vi "New 4ch.vi"(0 "VISA resource name out":refnum<visa-resource-name>, 9 "Number of channels":i32, 11 "error out":errorcluster) -> (3 "VISA resource name out 2":refnum<visa-resource-name>, 4 "element":dbl, 6 "element 2":dbl, 8 "element 3":dbl, 10 "element 4":dbl, 15 "error out 2":errorcluster)   [LabVIEW 2015]
uses:
  <instrlib>/Keithley 27XX/Public/Data/Read Multiple Direct.vi
  <instrlib>/Keithley 27XX/Keithley 27XX.lvlib
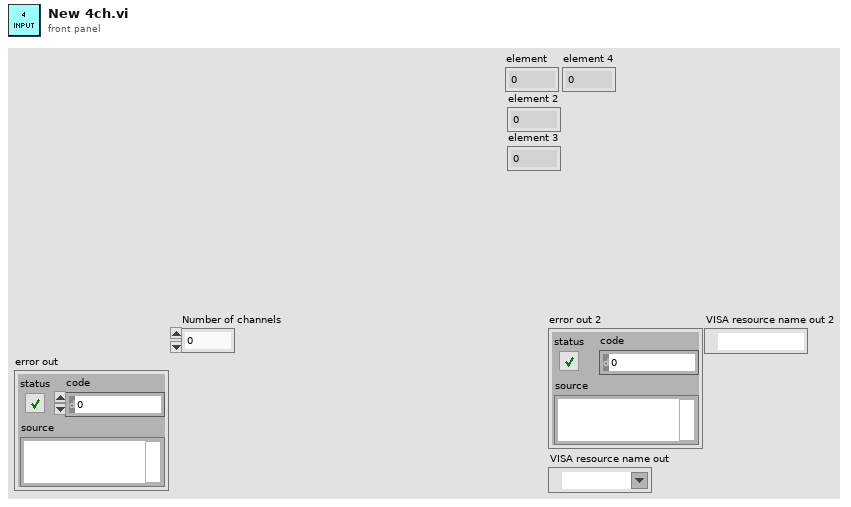
[diagram p1: front panel]
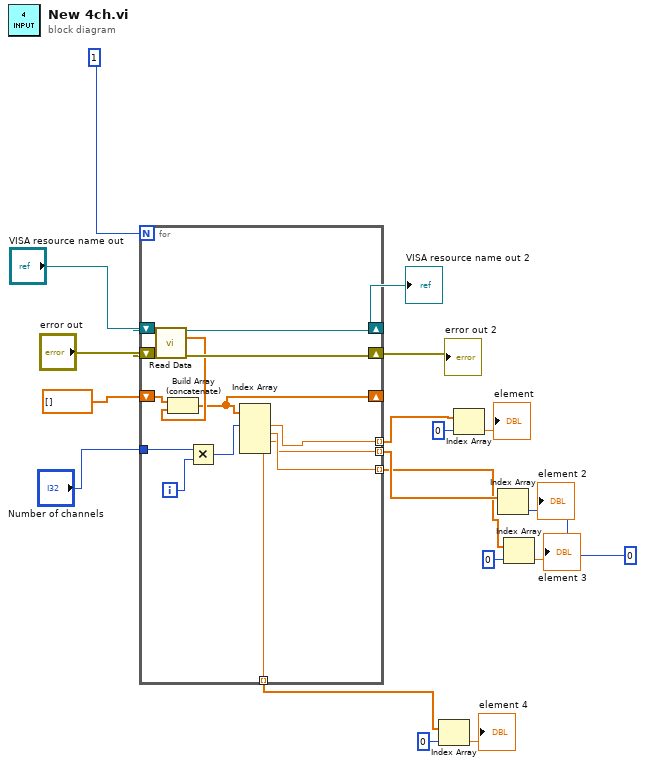
[diagram p0: block diagram]
diagram:
  n1 = for {
    N: 1 -> [_]
    shift-right: [w32] -> w18
    shift-left: "VISA resource name out" -> [w31]
    shift-right: [w33] -> w19
    shift-left: "error out" -> [w30]
    shift-right: [w24] -> _
    shift-left: dbl[] [] -> [w29]
    tunnel: "Number of channels" -> [w26]
    tunnel: [w23] -> w10 mode=indexing
    tunnel: [w22] -> w5 mode=indexing
    tunnel: [w21] -> w6 mode=indexing
    tunnel: [w20] -> w4 mode=indexing
    i -> [w27]
    n2 = call-poly <instrlib>:"Read Data.vi"("VISA resource name"=w31, "error in (no error)"=w30) -> ("VISA resource name out"=w32:refnum<visa-resource-name>, "Measurement Data"=w28:dbl[], "error out"=w33:errorcluster)  [unwired: 8 in, 3 out]
    n3 = Build Array (concatenate)(w29, w28) -> (w24:dbl[])
    n4 = Multiply(x=w26, y=w27) -> (x*y=w25:i32)
    n5 = Index Array(array=w24, index #1=w25) -> (element #1=w23:dbl, element #2=w22:dbl, element #3=w21:dbl, element #4=w20:dbl)  [unwired: 3 in]
  }
  "error out 2" <- w19
  "VISA resource name out 2" <- w18
  n6 = Index Array(array=w4, index=0) -> (element=→"element 4":dbl)
  n7 = Index Array(array=w10, index=0) -> (element=→"element":dbl)
  n8 = Index Array(array=w6, index=0) -> (element=→"element 2":dbl)
  n9 = Index Array(array=w5, index=0) -> (element=→"element 3":dbl)
